vi "Find SR in List.vi"(8 "new SR":T1 {"Creation Date" format="%<%x>T"; "Last Updated" format="%<%x>T"}, 11 "SR list in":T1[](array[typedef]) {"Creation Date" format="%<%x>T"; "Last Updated" format="%<%x>T"}) -> (0 "SR Index":i32, 1 "Is SR in List?":bool)   [LabVIEW 2018]
uses:
  Type Defs/SR Cluster.ctl
  Type Defs/SR Status.ctl
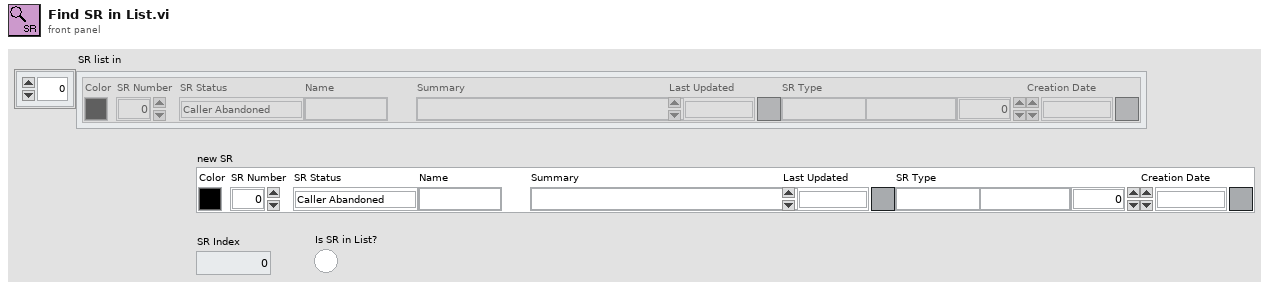
[diagram p1: front panel]
types:
  T1 = typedef "SR Cluster.ctl" = cluster{"Color":u32, "SR Number":i32, "SR Status":T2, "Name":string, "Summary":string, "Last Updated":timestamp, "SR Type":string, "Service Level":string, "Days Open":dbl, "Creation Date":timestamp}
  T2 = typedef "SR Status.ctl" = enum16{"Caller Abandoned", "Created in Error", "Expired", "Forum Resolved AE", "Forum Resolved Customer", "IN WORK", "IN WORK Collab with AES", "IN WORK Collab with PSE", "IN WORK Collab with SE", "IN WORK Customer Added Note", "IN WORK Escalation", "IN WORK Wait on Customer", "Open", "Potentially Resolved", "Presumed Resolved", "RMA Approved for Return", "Resolved", "Passed Off"}
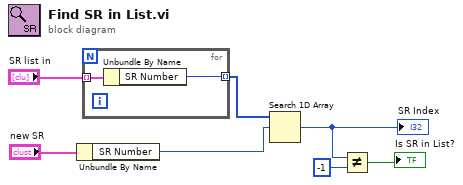
[diagram p0: block diagram]
diagram:
  n1 = Unbundle By Name("new SR") -> ("SR Number"=w4:i32)
  n2 = for {
    tunnel: "SR list in" -> [w9] mode=indexing
    tunnel: [w8] -> w5 mode=indexing
    n3 = Unbundle By Name(w9) -> ("SR Number"=w8:i32)
  }
  n4 = Search 1D Array(1D array=w5, element=w4) -> (index of element=w3:i32)  [unwired: 1 in]
  "SR Index" <- w3
  n5 = Not Equal?(x=w3, y=-1) -> (x != y?=→"Is SR in List?":bool)
